vi "initialize.vi"(8 "error in (no error)":errorcluster, 10 "action configuration":refnum<class "action configuration.lvclass">, 11 "Template Action Runtime in":refnum<class "Template Action Runtime.lvclass">) -> (0 "error out":errorcluster, 2 "data allocations":T1, 3 "Template Action Runtime out":refnum<class "Template Action Runtime.lvclass">)   [LabVIEW 2014, in "Template Action Runtime.lvclass"]
uses:
  Template Action Runtime.lvclass
  <vilib>/NI/TBM Modules/Sequencer/sequencer parent classes/action configuration parent/action configuration.lvclass
  <vilib>/NI/Tag Bus Module Framework/channel/data tables.ctl
  <vilib>/NI/Tag Bus/dictionary/data dictionary.lvclass
  <vilib>/NI/Tag Bus/dictionary table pair.ctl
  <vilib>/NI/Tag Bus/table/data table.ctl
  configuration/Template Action Cfg.lvclass
  configuration/Template Action Cfg.lvclass/Template Action Cfg.ctl
  Template Action Runtime.lvclass/Template Action Runtime.ctl
  <vilib>/NI/TBM Modules/Sequencer/sequencer parent classes/action parent/action.lvclass
  <vilib>/NI/Tag Bus/table/data table.lvlib
  <vilib>/NI/Tag Bus/tag bus.lvlib
  <vilib>/NI/Tag Bus Module Framework/channel/TBM channel.lvclass
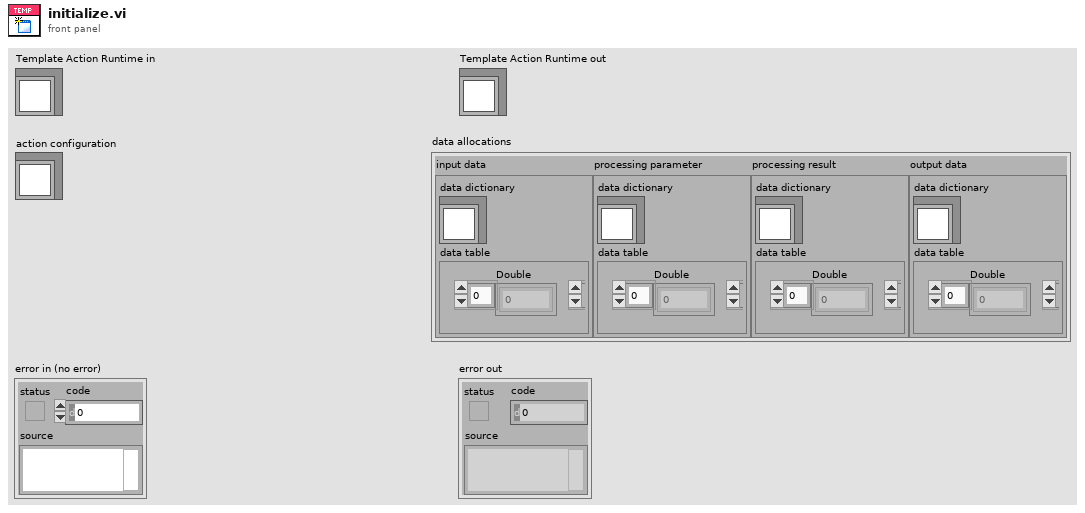
[diagram p1: front panel]
types:
  T1 = typedef "TBM channel.lvclass/data tables.ctl" = cluster{"input data":T2, "processing parameter":T2, "processing result":T2, "output data":T2}
  T2 = typedef "tag bus.lvlib/dictionary table pair.ctl" = cluster{"data dictionary":refnum<class "data dictionary.lvclass">, "data table":T3}
  T3 = typedef "tag bus.lvlib/data table.lvlib/data table.ctl" = cluster{"Double":dbl[], "Single":sgl[], "I64":i64[], "I32":i32[], "I16":i16[], "I8":i8[], "U64":u64[], "U32":u32[], "U16":u16[], "U8":u8[], "Boolean":bool[], "String":string[], "Array of Double":cluster{"DBL Array":dbl[]}[], "Array of Single":cluster{"SGL Array":sgl[]}[], "Array of I64":cluster{"I64 Array":i64[]}[], "Array of I32":cluster{"I32 Array":i32[]}[], "Array of I16":cluster{"I16 Array":i16[]}[], "Array of I8":cluster{"I8 Array":i8[]}[], "Array of U64":cluster{"U64 Array":u64[]}[], "Array of U32":cluster{"U32 Array":u32[]}[], "Array of U16":cluster{"U16 Array":u16[]}[], "Array of U8":cluster{"U8 Array":u8[]}[], "Array of Boolean":cluster{"Boolean Array":bool[]}[], "Array of String":cluster{"String Array":string[]}[]}
  T4 = typedef "Template Action Cfg.lvclass/configuration data.ctl" = cluster{"Placeholder":dbl}
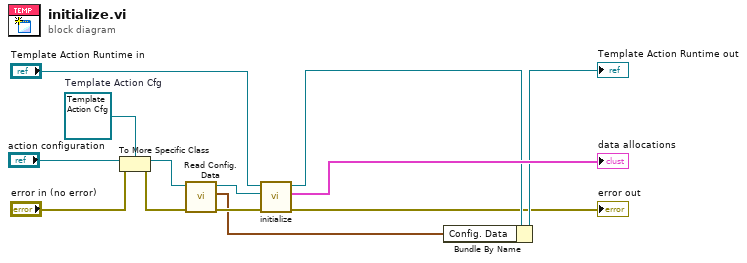
[diagram p0: block diagram]
diagram:
  w2 = refnum<class "Template Action Cfg.lvclass"> refnum  # Template Action Cfg
  n1 = To More Specific Class(target class=w2, reference="action configuration", error in="error in (no error)") -> (specific class reference=w6:refnum<class "Template Action Cfg.lvclass">, error out=w4:errorcluster)
  n2 = call "Read Config. Data.vi"("error in (no error)"=w4, "Template Action Cfg in"=w6) -> ("error out"=w8:errorcluster, "Config. Data"=w7:T4, "Template Action Cfg out"=w3:refnum<class "Template Action Cfg.lvclass">)  [unwired: 7 in]
  n3 = call-parent "initialize.vi"("error in (no error)"=w8, "action configuration"=w3, "Action in"="Template Action Runtime in") -> ("error out"=→"error out":errorcluster, "data allocations"=→"data allocations":T1, "Action out"=w11:refnum<class "Template Action Runtime.lvclass">)  [unwired: 6 in]
  n4 = Bundle By Name(cluster=w11, "Config. Data"=w7) -> (→"Template Action Runtime out":refnum<class "Template Action Runtime.lvclass">)
